vi "Rysowanie planszy.vi"(11 "Array in":dbl[][](array[numeric])) -> (3 "Array out":u32[][](array[numeric]))   [LabVIEW 2020]
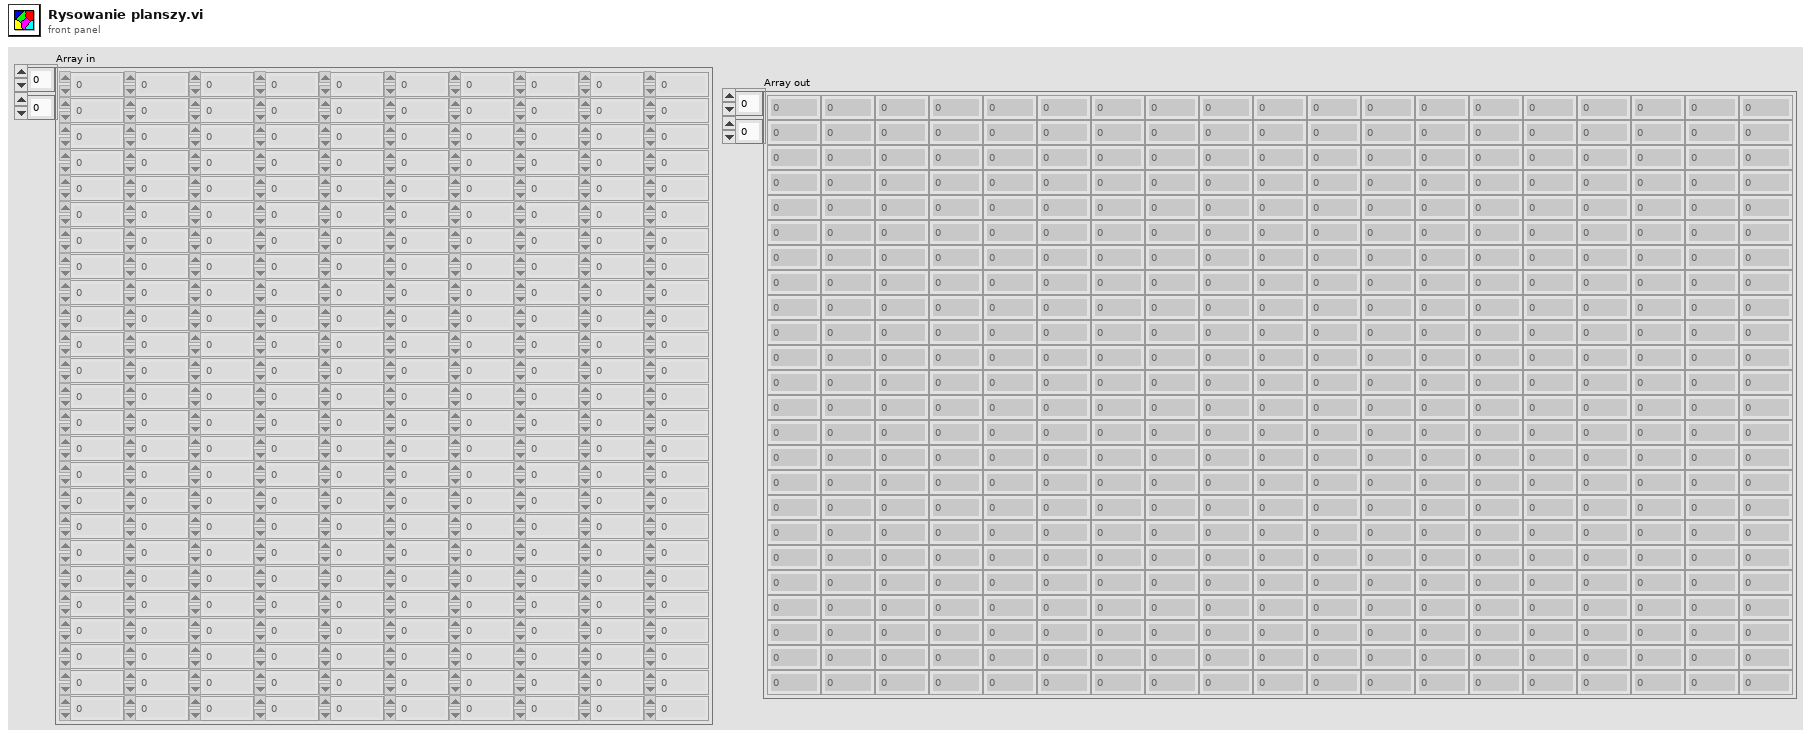
[diagram p1: front panel]
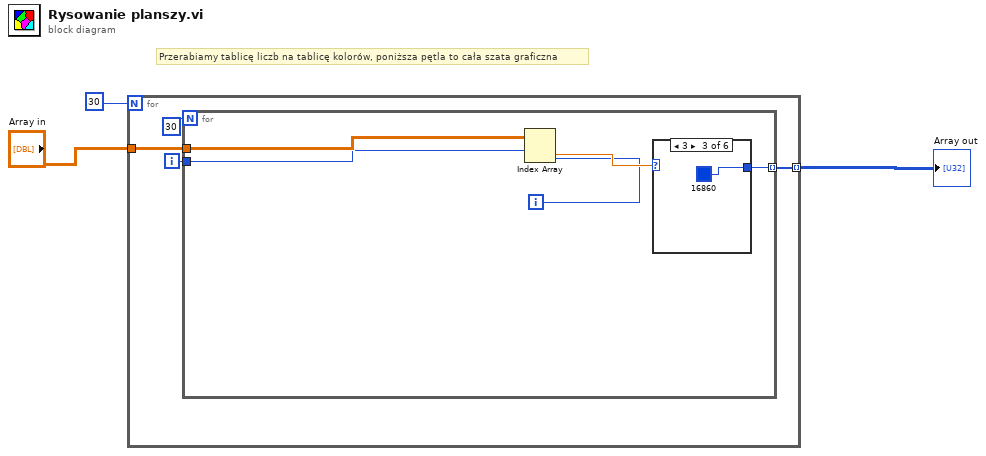
[diagram p0: block diagram]
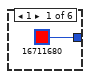
[diagram p2: hidden frame]
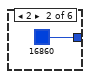
[diagram p3: hidden frame]
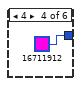
[diagram p4: hidden frame]
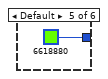
[diagram p5: hidden frame]
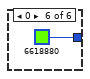
[diagram p6: hidden frame]
diagram:
  # "Przerabiamy tablicę liczb na tablicę kolorów, poniższa pętla to cała szata graficzna"
  n1 = for {
    N: 30 -> [_]
    tunnel: "Array in" -> [w7]
    tunnel: [w4] -> w1 mode=indexing
    i -> [w5]
    n2 = for {
      N: 30 -> [_]
      tunnel: w7 -> [w12]
      tunnel: w5 -> [w9]
      tunnel: [w8] -> w4 mode=indexing
      i -> [w10]
      n3 = Index Array(array=w12, index (row)=w9, index (col)=w10) -> (element=w11:dbl)
      n4 = case shown="3" w11 {
        tunnel: [u32 16711680 u32 16860 u32 16860 u32 16711912 u32 6618880 u32 6618880] -> w8
        frame 1 {
        }
        frame 2 {
        }
        frame 3 {
        }
        frame 4 {
        }
        frame Default {
        }
        frame 0 {
        }
      }
    }
  }
  "Array out" <- w1
